vi "Mother_doc.vi"() -> ()   [LabVIEW 2021]
uses:
  <vilib>/Utility/file.llb/Write Delimited Spreadsheet (DBL).vi
panel:
  in  "Estimated Length (mm)":dbl
  in  "Estimated Width (mm)":dbl
  out "Double - Voltage":dbl
  out "Double - Current":dbl
  out "First Cycle Reverse Sweep":cluster{"Y":dbl[], "Y":dbl[]}[](graph)
  out "First Cycle Forward Sweep":cluster{"Y":dbl[], "Y":dbl[]}[](graph)
  out "Single - Current":dbl
  out "Single - Voltage":dbl
  out "Recorded_Data":dbl[][][](array[numeric])
  out "WarmUp":dbl[][](array[numeric])
  out "Values Committed":bool
  in  "Press to start":bool
  in  "Set Swe_2_Mode":string(combo)="Single"
  in  "Set Swe_1_Mode":string(combo)="Single"
  in  "SMU1 Terminal":string(combo)="Source"
  in  "Sample Information":string="Made_up"
  in  "User":string="Richard"
  out "error out":errorcluster
  in  "VISA resource name":refnum<visa-resource-name>="PA"
  out "DorG_2":string
  out "DorG_1":string
  in  "VIntegration_2":dbl=100.0
  in  "VIntegration_1":dbl=100.0
  out "V_Cst_2 [V]":dbl
  out "V Cst_1 [V]":dbl
  out "V Cst_0 [V]":dbl
  out "V Step_2":dbl
  out "V Step_1":dbl
  out "V Step_0":dbl
  in  "Vvar_2_points":dbl=10.0
  in  "Vvar_1_points":dbl=10.0
  in  "Vvar_0_points":dbl=10.0
  in  "DorG_0":string(combo)="Gate"
  in  "Vvar_2_Stop":dbl=1.0
  in  "Vvar_1_Stop":dbl=1.0
  in  "Vvar_0_Stop":dbl
  in  "Vvar_2_start":dbl
  in  "Vvar_1_start":dbl
  in  "Vvar_0_start":dbl
  in  "# Cycles":dbl=1.0
  in  "Sweep Spacing_2":string(combo)="Linear"
  in  "Sweep Spacing_1":string(combo)="Linear"
  in  "Sweep Spacing_0":string(combo)="Linear"
  in  "VIntegration_0":dbl=100.0
  in  "Gate Current Compliance 2":dbl=1e-06
  in  "Gate Current Compliance 1":dbl=1e-06
  in  "Gate Current Compliance 0":dbl=1e-06
  in  "Drain Current Compliance 2":dbl=0.0001 format="%#_6p"
  in  "Drain Current Compliance 1":dbl=0.01 format="%#_6p"
  in  "Drain Current Compliance":dbl=1e-06
  in  "Sweep 2":bool
  in  "Sweep 0":bool
  in  "Vvar-2_delaytime":dbl
  in  "Vvar_1_delaytime":dbl
  in  "Vvar-0_delaytime":dbl
  in  "Vvar_2_holdtime":dbl
  in  "Vvar_1_holdtime":dbl
  in  "Vvar_0_holdtime":dbl
  out "VISA resource name out":refnum<visa-resource-name>
  in  "error in (no error)":errorcluster
  out "SMU3 Terminal":string
  out "SMU2 Terminal":string
  out "Sweep 2 Point Checker":string
  out "Sweep 2 Pot Check":string
  out "Sweep 1 Point Checker":string
  out "Sweep 1 Pot Check":string
  out "Gate Point number Checker":string
  out "Gate Potential_checker":string
  in  "V_const_2":dbl
  in  "V_const_1":dbl
  in  "V_const_0":dbl
  in  "Vstep2":dbl
  in  "Vstep1":dbl
  in  "Vstep0":dbl
  # "Meta Data"
  # "I(S)"
  # "I(G)"
  # "Voltage"
  # "T(G)"
  # "T(S)"
  # "T(D)"
  # "I(D)"
  # "Warmup is not yet fully implemented"
  # "V Stop"
  # "Sweep Mode"
  # "Delay Time"
  # "Drain/Gate"
  # "V Start"
  # "# Points"
  # "V Step"
  # "V Cst"
  # "Sweep Spacing"
  # "Drain Current Comp"
  # "Gate Current Comp"
  # "Hold Time"
  # "Integration"
  # "Single"
  # "V Stop"
  # "Sweep Mode"
  # "Delay Time"
  # "Drain/Gate"
  # "V Start"
  # "# Points"
  # "V Step"
  # "V Cst"
  # "Sweep Spacing"
  # "Drain Current Comp"
  # "Gate Current Comp"
  # "Hold Time"
  # "Integration"
  # "Operational_placeholders do not modify"
  # "Second_sweep is not yet implemented"
  # "V Stop"
  # "Sweep Mode"
  # "Delay Time"
  # "Drain/Gate"
  # "V Start"
  # "# Points"
  # "V Step"
  # "V Cst"
  # "Sweep Spacing"
  # "Drain Current Comp"
  # "Gate Current Comp"
  # "Hold Time"
  # "Integration"
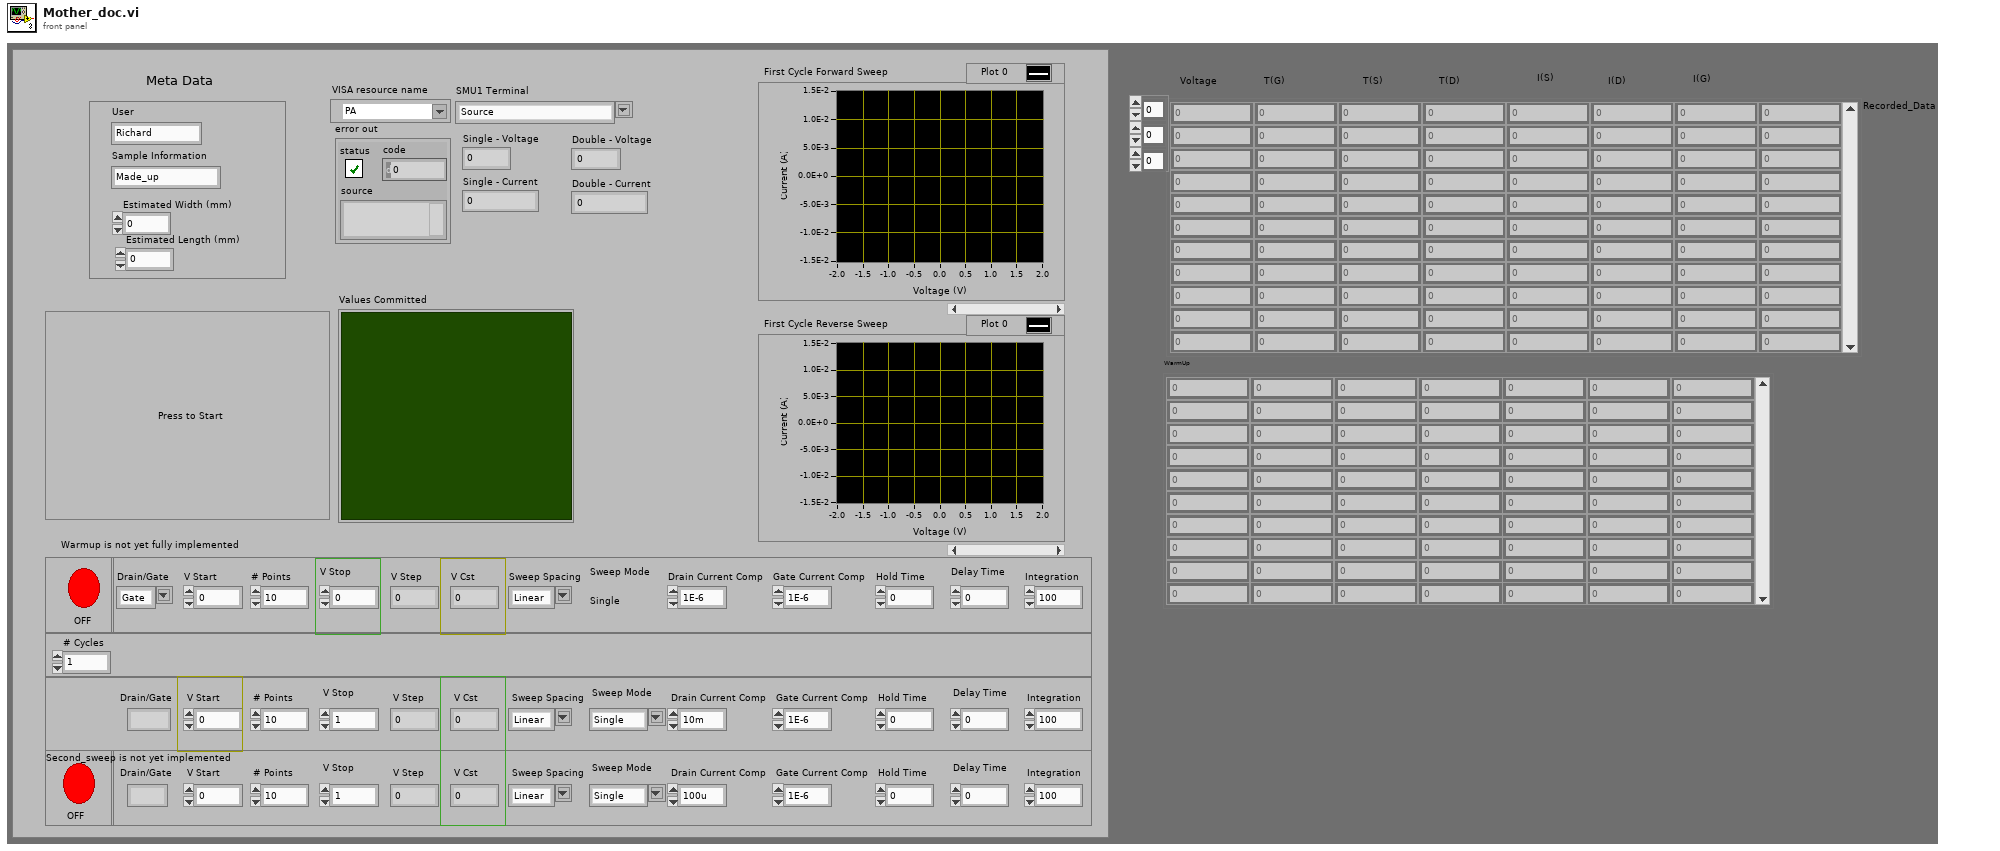
[diagram p1: front panel]
types:
  T1 = enum16{"open", "replace", "create", "open or create", "replace or create", "replace or create with confirmation"}
  T2 = cluster{"DorG_0":string, "Vvar_0_start":dbl, "Vstep0":dbl, "Vvar_0_Stop":dbl, "V_const_0":dbl, "Drain Current Compliance":dbl, "Gate Current Compliance 0":dbl, "Vvar_0_holdtime":dbl, "Vvar-0_delaytime":dbl, "Output Integration":dbl, string, "Sweep Spacing_0":string}
  T3 = cluster{string, "Vvar_1_start ":dbl, "Vstep1":dbl, "Vvar_1_Stop":dbl, "V_const_1":dbl, "Drain Current Compliance 1":dbl, "Gate Current Compliance 1":dbl, "Vvar_1_holdtime":dbl, "Vvar_1_delaytime":dbl, "Output Integration":dbl, "Set Swe_1_Mode":string, "Sweep Spacing_1":string}
  T4 = cluster{string, "Vvar_2_start":dbl, "Vstep2":dbl, "Vvar_2_Stop":dbl, "V_const_2":dbl, "Drain Current Compliance 2":dbl, "Gate Current Compliance 2":dbl, "Vvar_2_holdtime":dbl, "Vvar-2_delaytime":dbl, "Output Integration":dbl, "Set Swe_2_Mode":string, "Sweep Spacing_2":string}
  T5 = cluster{"DorG":string, "Vvar_start":dbl, "Vvar_step":dbl, "Vvar_Stop":dbl, "V_const ":dbl, "Drain Current Compliance":dbl, "Gate Current Compliance":dbl, "Vvar_holdtime":dbl, "Vvar_delaytime":dbl, "IntPts":dbl, "Set Swe_Mode":string, "Sweep Spacing":string}
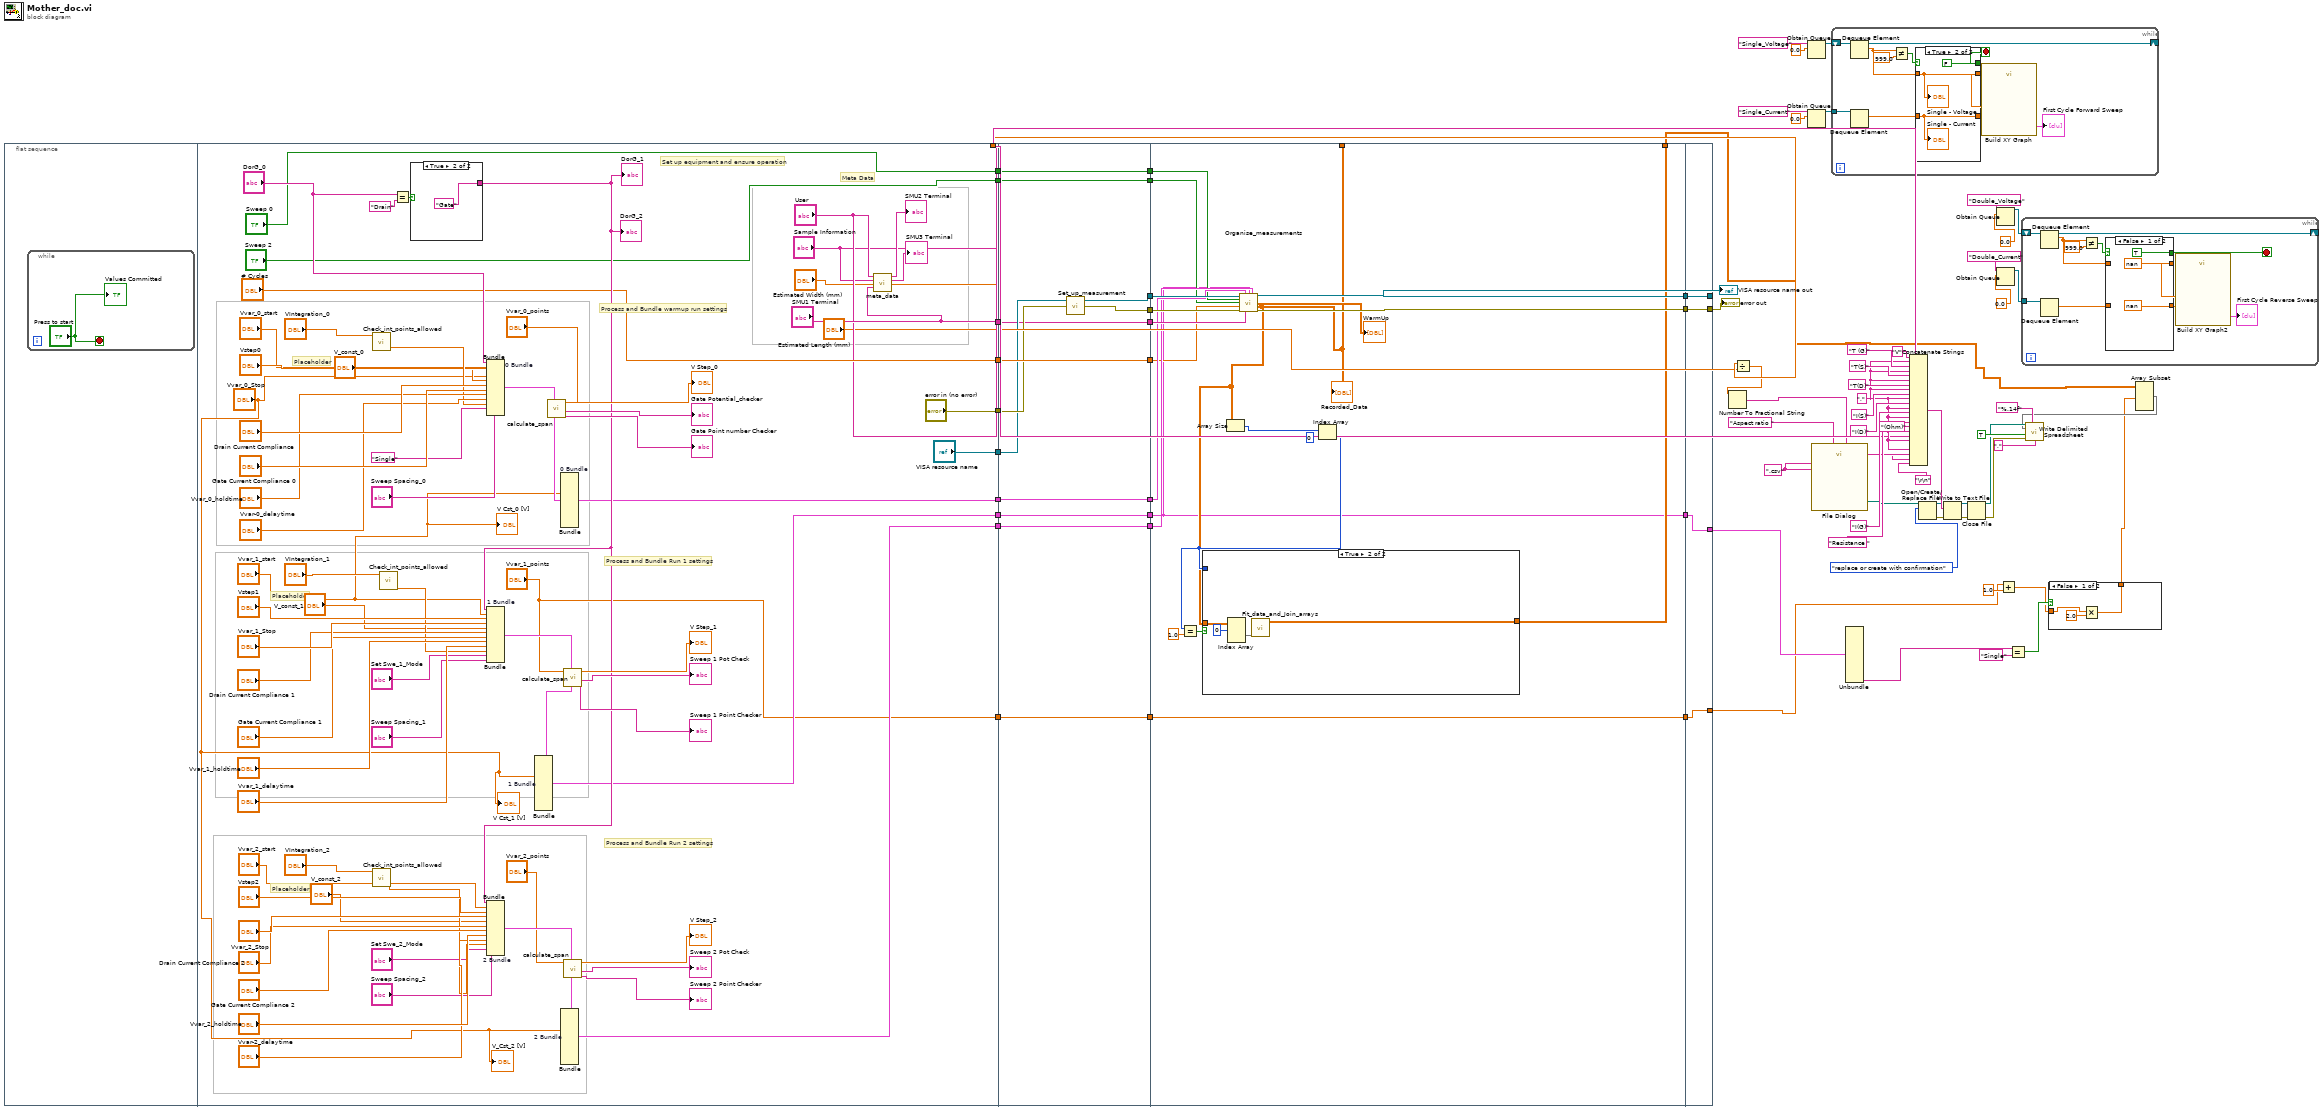
[diagram p0: block diagram]
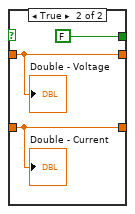
[diagram p3: hidden frame]
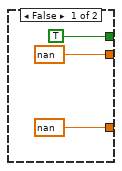
[diagram p4: hidden frame]
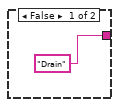
[diagram p5: hidden frame]
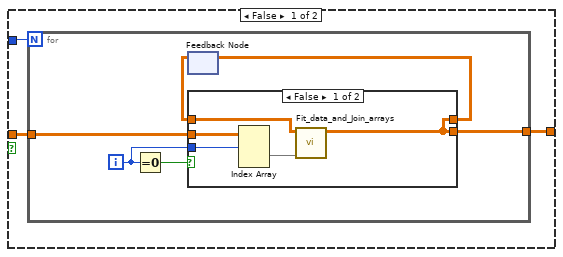
[diagram p6: hidden frame]
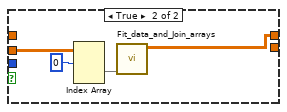
[diagram p7: hidden frame]
diagram:
  w30 = "," ("string")
  w39 = ".csv" ("pattern (all files)")
  n1 = flat-sequence {
    tunnel: ["# Cycles"] -> w77
    tunnel: ["error in (no error)"] -> w73
    tunnel: ["VISA resource name"] -> w72
    tunnel: ["SMU1 Terminal"] -> w71
    tunnel: [w91] -> w69
    tunnel: [w90] -> w67
    tunnel: [w89] -> w65
    tunnel: ["Sweep 2"] -> w63
    tunnel: ["Sweep 0"] -> w61
    tunnel: ["User"] -> w29
    tunnel: ["Sample Information"] -> w28
    tunnel: ["Estimated Width (mm)"] -> w20
    tunnel: ["Estimated Length (mm)"] -> w19
    tunnel: ["Vvar_1_points"] -> w5
    tunnel: w77 -> [w167]
    tunnel: [w167] -> w76
    tunnel: [w166] -> w75
    tunnel: [w165] -> w74
    tunnel: w73 -> [w164]
    tunnel: w72 -> [w163]
    tunnel: w71 -> [w162]
    tunnel: [w162] -> w70
    tunnel: w69 -> [w161]
    tunnel: [w161] -> w68
    tunnel: w67 -> [w160]
    tunnel: [w160] -> w66
    tunnel: w65 -> [w159]
    tunnel: [w159] -> w64
    tunnel: w63 -> [w158]
    tunnel: [w158] -> w62
    tunnel: w61 -> [w157]
    tunnel: [w157] -> w60
    tunnel: [w156] -> w6
    tunnel: w5 -> [w156]
    tunnel: w76 -> [w170]
    tunnel: w75 -> [w185]
    tunnel: w74 -> [w184]
    tunnel: w70 -> [w183]
    tunnel: w68 -> [w182]
    tunnel: w66 -> [w169]
    tunnel: w64 -> [w181]
    tunnel: w62 -> [w180]
    tunnel: w60 -> [w179]
    tunnel: [w187] -> w59
    tunnel: [w186] -> w58
    tunnel: [w172] -> w14
    tunnel: [w171] -> _
    tunnel: [w169] -> w12
    tunnel: w6 -> [w168]
    tunnel: [w168] -> w4
    tunnel: [w212] -> w78
    tunnel: [w213] -> w79
    tunnel: w59 -> [w213]
    tunnel: w58 -> [w212]
    tunnel: w12 -> [w211]
    tunnel: [w211] -> w11
    tunnel: w4 -> [w210]
    tunnel: [w210] -> w2
    frame #0 {
      n2 = while {
        stop <- "Press to start" stop-if-true
        "Values Committed" <- "Press to start"
      }
    }
    frame #1 {
      # "Set up equipment and ensure operation"
      # "Meta Data"
      # "Process and Bundle warmup run settings"
      # "Process and Bundle Run 1 settings"
      # "Process and Bundle Run 2 settings"
      # "Placeholder"
      # "Placeholder"
      # "Placeholder"
      n3 = call "Check_int_points_allowed.vi"("Integration Points"="VIntegration_0") -> ("Output Integration"=w135:dbl)  [unwired: 9 in, 1 out]
      n4 = call "Check_int_points_allowed.vi"("Integration Points"="VIntegration_2") -> ("Output Integration"=w105:dbl)  [unwired: 9 in, 1 out]
      n5 = call "Check_int_points_allowed.vi"("Integration Points"="VIntegration_1") -> ("Output Integration"=w118:dbl)  [unwired: 9 in, 1 out]
      n6 = Equal?(x="DorG_0", y="Drain") -> (x = y?=w151:bool)
      n7 = case shown="True" w151 {
        tunnel: ["Drain" "Gate"] -> w115
        frame False {
        }
        frame True {
        }
      }
      "DorG_1" <- w115
      "DorG_2" <- w115
      n8 = Bundle "0 Bundle"("DorG_0"="DorG_0", "Vvar_0_start"="Vvar_0_start", "Vstep0"="Vstep0", "Vvar_0_Stop"="Vvar_0_Stop", "V_const_0"="V_const_0", "Drain Current Compliance"="Drain Current Compliance", "Gate Current Compliance 0"="Gate Current Compliance 0", "Vvar_0_holdtime"="Vvar_0_holdtime", "Vvar-0_delaytime"="Vvar-0_delaytime", "Output Integration"=w135, "Single", "Sweep Spacing_0"="Sweep Spacing_0") -> (w129:T2)  [unwired: 1 in]
      n9 = Bundle "1 Bundle"(w115, "Vvar_1_start"="Vvar_1_start", "Vstep1"="Vstep1", "Vvar_1_Stop"="Vvar_1_Stop", "V_const_1"="V_const_1", "Drain Current Compliance 1"="Drain Current Compliance 1", "Gate Current Compliance 1"="Gate Current Compliance 1", "Vvar_1_holdtime"="Vvar_1_holdtime", "Vvar_1_delaytime"="Vvar_1_delaytime", "Output Integration"=w118, "Set Swe_1_Mode"="Set Swe_1_Mode", "Sweep Spacing_1"="Sweep Spacing_1") -> (w125:T3)  [unwired: 1 in]
      n10 = Bundle "2 Bundle"(w115, "Vvar_2_start"="Vvar_2_start", "Vstep2"="Vstep2", "Vvar_2_Stop"="Vvar_2_Stop", "V_const_2"="V_const_2", "Drain Current Compliance 2"="Drain Current Compliance 2", "Gate Current Compliance 2"="Gate Current Compliance 2", "Vvar_2_holdtime"="Vvar_2_holdtime", "Vvar-2_delaytime"="Vvar-2_delaytime", "Output Integration"=w105, "Set Swe_2_Mode"="Set Swe_2_Mode", "Sweep Spacing_2"="Sweep Spacing_2") -> (w113:T4)  [unwired: 1 in]
      n11 = call "calculate_span.vi"("Sweep in"=w129, "V_points"="Vvar_0_points") -> ("Gate Point number Checker"=→"Gate Point number Checker":string, "Gate Potential_checker"=→"Gate Potential_checker":string, "V Step"=→"V Step_0":dbl, "Sweep out"=w128:T5)  [unwired: 6 in]
      n12 = Bundle "0 Bundle"(cluster=w128, "V_const"="Vvar_1_start") -> (w91:T5)  [unwired: 11 in]
      n13 = call "calculate_span.vi"("Sweep in"=w125, "V_points"="Vvar_1_points") -> ("Gate Point number Checker"=→"Sweep 1 Point Checker":string, "Gate Potential_checker"=→"Sweep 1 Pot Check":string, "V Step"=→"V Step_1":dbl, "Sweep out"=w124:T5)  [unwired: 6 in]
      n14 = Bundle "1 Bundle"(cluster=w124, "V_const"="Vvar_0_Stop") -> (w90:T5)  [unwired: 11 in]
      n15 = call "calculate_span.vi"("Sweep in"=w113, "V_points"="Vvar_2_points") -> ("Gate Point number Checker"=→"Sweep 2 Point Checker":string, "Gate Potential_checker"=→"Sweep 2 Pot Check":string, "V Step"=→"V Step_2":dbl, "Sweep out"=w112:T5)  [unwired: 6 in]
      n16 = Bundle "2 Bundle"(cluster=w112, "V_const"="Vvar_0_Stop") -> (w89:T5)  [unwired: 11 in]
      n17 = call "meta_data.vi"("User"="User", "Sample Information"="Sample Information", "SMU1 Terminal"="SMU1 Terminal") -> ("SMU2 Terminal"=→"SMU2 Terminal":string, "SMU3 Terminal"=→"SMU3 Terminal":string)  [unwired: 11 in]
      "V Cst_0 [V]" <- "Vvar_1_start"
      "V Cst_1 [V]" <- "Vvar_0_Stop"
      "V_Cst_2 [V]" <- "Vvar_0_Stop"
    }
    frame #2 {
      n18 = call "Set_up_measurement.vi"("error in (no error)"=w164, "VISA resource name"=w163) -> ("error out"=w166:errorcluster, "VISA resource name out"=w165:refnum<visa-resource-name>)  [unwired: 2 in]
    }
    frame #3 {
      n19 = call "Organise_measurements.vi"("VISA resource name"=w184, 1:"Sweep 0"=w182, "Sweep 1_replac"=w169, "Sweep 2_replac 2"=w181, 5:"Sweep 0"=w179, "Sweep 2"=w180, "# Cycles"=w170, "error in (no error)"=w185, "SMU1 Terminal"=w183) -> ("VISA resource name out"=w187:refnum<visa-resource-name>, "WarmUp"=→"WarmUp":dbl[][], "Recorded_Data"=w171:dbl[][][], "error out"=w186:errorcluster)  [unwired: 3 in]
      "Recorded_Data" <- w171
      n20 = Array Size(array=w171) -> (size(s)=w177:i32[])
      n21 = Index Array(array=w177, index=0) -> (element=w173:i32)
      n22 = Equal?(x=w173, y=1.0) -> (x = y?=w174:bool)
      n23 = case shown="True" w174 {
        tunnel: w171 -> [w189 w208]
        tunnel: [w188 w206] -> w172
        tunnel: w173 -> [w190 _]
        frame False {
          n24 = for {
            N: w190 -> [_]
            tunnel: w189 -> [w195]
            tunnel: [w191] -> w188
            i -> [w192]
            n25 = Equal To 0?(x=w192) -> (x = 0?=w196:bool)
            n26 = feedback #1() -> (w193:dbl[][])  [unwired: 1 in]
            n27 = case shown="False" w196 {
              tunnel: w195 -> [w200 w205]
              tunnel: [w197 w202] -> w194
              tunnel: w193 -> [w201 _]
              tunnel: w192 -> [w199 _]
              tunnel: [w197 _] -> w191
              frame False {
                n28 = Index Array(array=w200, index (dim 0)=w199) -> (element=w198:dbl[][])  [unwired: 2 in]
                n29 = call "Fit_data_and_Join_arrays.vi"("Array to be added"=w198, "Old Array"=w201) -> ("Output array"=w197:dbl[][])  [unwired: 9 in]
              }
              frame True {
                n30 = Index Array(array=w205, index (dim 0)=0 ("index (page)")) -> (element=w203:dbl[][])  [unwired: 2 in]
                n31 = call "Fit_data_and_Join_arrays.vi"("Array to be added"=w203) -> ("Output array"=w202:dbl[][])  [unwired: 10 in]
              }
            }
            n32 = feedback-in #1(w194) -> ()
          }
        }
        frame True {
          n33 = Index Array(array=w208, index (dim 0)=0 ("index (page)")) -> (element=w207:dbl[][])  [unwired: 2 in]
          n34 = call "Fit_data_and_Join_arrays.vi"("Array to be added"=w207) -> ("Output array"=w206:dbl[][])  [unwired: 10 in]
        }
      }
    }
    frame #4 {
    }
  }
  n35 = Divide(x=w20, y=w19) -> (x/y=w15:dbl)
  n36 = Number To Fractional String(number=w15) -> (F-format string=w16:string)  [unwired: 3 in]
  n37 = Obtain Queue(name (unnamed)="Single_Voltage", element data type=0.0) -> (queue out=w55:refnum<queue>)  [unwired: 3 in, 2 out]
  n38 = Obtain Queue(name (unnamed)="Single_Current", element data type=0.0) -> (queue out=w52:refnum<queue>)  [unwired: 3 in, 2 out]
  n39 = call "File Dialog"("pattern (all files)"=w39, "pattern label"=w39) -> ("selected path"=w38:path)  [unwired: 10 in, 3 out]
  n40 = while {
    shift-right: [w223] -> _
    shift-left: w55 -> [w224]
    tunnel: w52 -> [w218]
    stop <- w222 stop-if-true
    n41 = Dequeue Element(queue=w224) -> (queue out=w223:refnum<queue>, element=w220:dbl)  [unwired: 2 in, 2 out]
    n42 = Dequeue Element(queue=w218) -> (element=w217:dbl)  [unwired: 2 in, 3 out]
    n43 = Not Equal?(x=w220, y=999.0) -> (x != y?=w219:bool)
    n44 = case shown="True" w219 {
      tunnel: w220 -> [_ w229]
      tunnel: [TRUE FALSE] -> w222
      tunnel: [nan w229] -> w215
      tunnel: w217 -> [_ w228]
      tunnel: [nan w228] -> w214
      frame False {
      }
      frame True {
        "Single - Voltage" <- w229
        "Single - Current" <- w228
      }
    }
    n45 = call "Build XY Graph"("Y Input"=w214, "X Input"=w215) -> ("XY Graph"=→"First Cycle Forward Sweep":cluster{"X":dbl[], "Y":dbl[]}[])  [unwired: 8 in, 1 out]
  }
  n46 = Unbundle(w11) -> ("Sweep Spacing"=w10:string)  [unwired: 11 out]
  n47 = Concatenate Strings("V" ("string"), w30, "T (G)" ("string"), w30, "T(S)" ("string"), w30, "T(D)" ("string"), w30, "I(S)" ("string"), w30, "I(D)" ("string"), w30, "I(G)" ("string"), w30, "Resistance " ("string"), "(Ohm)" ("string"), w30, w29, w30, w28, w30, "Aspect ratio " ("string"), w16, "\r\n") -> (w40:string)
  n48 = Open/Create/Replace File(file path (use dialog)=w38, operation (0:open)=T1."replace or create with confirmation") -> (refnum out=w33:refnum<file>, error out=w34:errorcluster)  [unwired: 4 in, 1 out]
  n49 = Write to Text File(file (use dialog)=w33, text=w40, error in=w34) -> (refnum out=w36:refnum<file>, error out=w35:errorcluster)  [unwired: 1 in, 1 out]
  n50 = Close File(refnum=w36, error in=w35) -> (path=w48:path, error out=w49:errorcluster)
  n51 = Obtain Queue(name (unnamed)="Double_Voltage", element data type=0.0) -> (queue out=w25:refnum<queue>)  [unwired: 3 in, 2 out]
  n52 = Obtain Queue(name (unnamed)="Double_Current", element data type=0.0) -> (queue out=w22:refnum<queue>)  [unwired: 3 in, 2 out]
  n53 = Add(x=w2, y=1.0) -> (x+y=w1:dbl)
  n54 = Equal?(x=w10, y="Single") -> (x = y?=w7:bool)
  n55 = while {
    shift-right: [w240] -> _
    shift-left: w25 -> [w241]
    tunnel: w22 -> [w235]
    stop <- w239 stop-if-true
    n56 = Dequeue Element(queue=w241) -> (queue out=w240:refnum<queue>, element=w237:dbl)  [unwired: 2 in, 2 out]
    n57 = Dequeue Element(queue=w235) -> (element=w234:dbl)  [unwired: 2 in, 3 out]
    n58 = Not Equal?(x=w237, y=999.0) -> (x != y?=w236:bool)
    n59 = case shown="False" w236 {
      tunnel: w237 -> [_ w246]
      tunnel: [TRUE FALSE] -> w239
      tunnel: [nan w246] -> w232
      tunnel: w234 -> [_ w245]
      tunnel: [nan w245] -> w231
      frame False {
      }
      frame True {
        "Double - Voltage" <- w246
        "Double - Current" <- w245
      }
    }
    n60 = call "Build XY Graph2"("Y Input"=w231, "X Input"=w232) -> ("XY Graph"=→"First Cycle Reverse Sweep":cluster{"X":dbl[], "Y":dbl[]}[])  [unwired: 8 in, 1 out]
  }
  n61 = case shown="False" w7 {
    tunnel: [w248 w251] -> w8
    tunnel: w1 -> [w249 w251]
    frame False {
      n62 = Multiply(x=w249, y=2.0) -> (x*y=w248:dbl)
    }
    frame True {
    }
  }
  n63 = Array Subset(array=w14, length (row)=w8) -> (w13:dbl[][])  [unwired: 3 in]
  n64 = call-poly <vilib>:"Write Delimited Spreadsheet.vi"("file path (dialog if empty)"=w48, "format (%.3f)"="%.14f", "2D data"=w13, "append to file? (new file:F)"=TRUE, "error in (no error)"=w49, "delimiter (\\t)"="," ("delimiter (\\t)")) -> ()  [unwired: 8 in, 2 out]
  "error out" <- w78
  "VISA resource name out" <- w79
